vi "Set System LED.vi"(0 "VISA resource name":refnum<visa-resource-name>, 5 "LED Blink (F: Disable)":bool, 11 "error in (no error)":errorcluster) -> (4 "VISA resource name out":refnum<visa-resource-name>, 15 "error out":errorcluster)   [LabVIEW 2012, in "NH Research Regenerative Test Series.lvlib"]
doc: "Causes the LED on the Module to blink."
uses:
  <instrlib>/NH Research Regenerative Test Series/NH Research Regenerative Test Series.lvlib
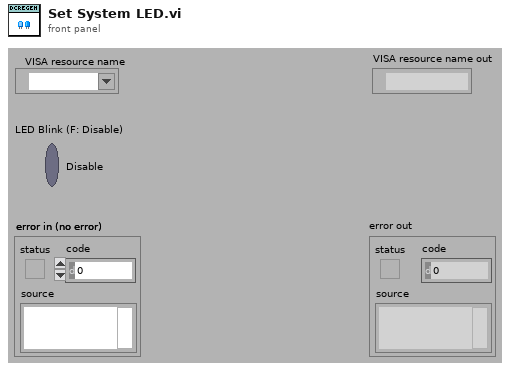
[diagram p1: front panel]
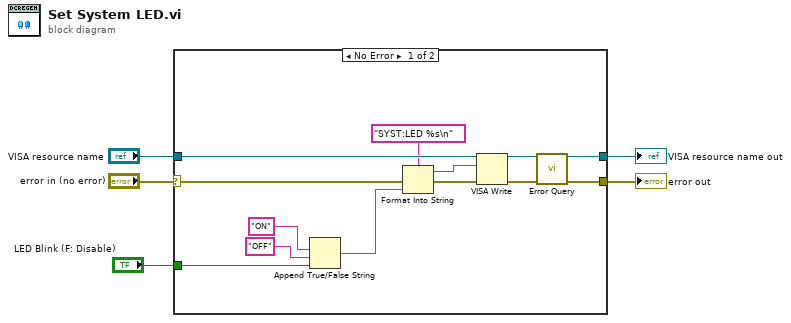
[diagram p0: block diagram]
diagram:
  n1 = case shown="No Error" "error in (no error)" {
    selector: "error in (no error)" -> [w13 w20]
    tunnel: "VISA resource name" -> [w18 w19]
    tunnel: [w17 w19] -> w4
    tunnel: [w16 w20] -> w3
    tunnel: "LED Blink (F: Disable)" -> [w7 _]
    frame No Error {
      n2 = Append True/False String(1:w7, 2:"OFF", 3:"ON") -> (0:w6:string)  [unwired: 1 in]
      n3 = Format Into String(format string="SYST:LED %s\n", error in=w13, w6) -> (resulting string=w10:string, error out=w11:errorcluster)  [unwired: 1 in]
      n4 = VISA Write(VISA resource name=w18, write buffer=w10, error in (no error)=w11) -> (VISA resource name out=w15:refnum<visa-resource-name>, error out=w14:errorcluster)  [unwired: 1 out]
      n5 = call <instrlib>:"Error Query.vi"("VISA resource name"=w15, "error in (no error)"=w14) -> ("VISA resource name out"=w17:refnum<visa-resource-name>, "error out"=w16:errorcluster)  [unwired: 10 in, 2 out]
    }
    frame Error {
    }
  }
  "error out" <- w3
  "VISA resource name out" <- w4
